vi "Conversion I16-14bits to DBL.vi"(4 "Array":i16[](array[numeric])) -> (1 "Array Out":dbl[](array[numeric]) format="%.6p")   [LabVIEW 2019]
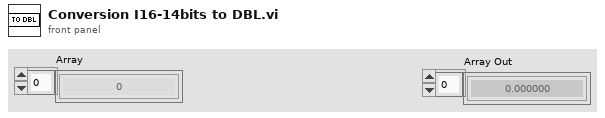
[diagram p1: front panel]
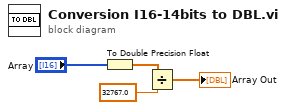
[diagram p0: block diagram]
diagram:
  n1 = To Double Precision Float(number="Array") -> (double precision float=w3:dbl[])
  n2 = Divide(x=w3, y=32767.0) -> (x/y=→"Array Out":dbl[])
